vi "Create Icon Framework.vi"(10 "Template Glyph":picture, 11 "Layer name":string) -> (3 "Icon Framework out":refnum<class "Icon Framework.lvclass">)   [LabVIEW 2020, in "LabVIEW Icon API.lvlib"]
doc: "Create the Icon Framework (Template or Text class) class."
uses:
  <vilib>/LabVIEW Icon API/LabVIEW Icon API.lvlib
  <vilib>/LabVIEW Icon API/lv_icon/Classes/Icon Framework/Icon Framework.lvclass
  <vilib>/LabVIEW Icon API/lv_icon/Controls/Layer.ctl
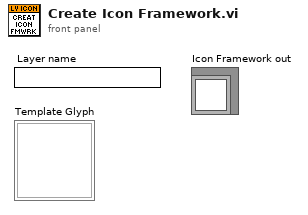
[diagram p1: front panel]
types:
  T1 = typedef "Layer.ctl" = cluster{"LayerIcon":picture, "LayerName":string, "Opacity":u8, "Visibility?":bool}
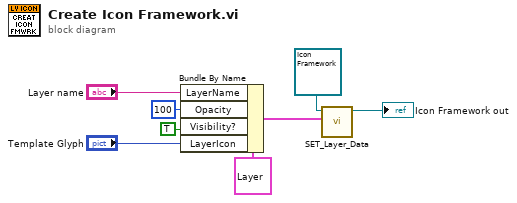
[diagram p0: block diagram]
diagram:
  n1 = Bundle By Name(cluster=T1 {"LayerIcon"=bytes[3102], "LayerName"="", "Opacity"=100, "Visibility?"=TRUE} ("Data"), "LayerName"="Layer name", "Opacity"=u8 100, "Visibility?"=TRUE, "LayerIcon"="Template Glyph") -> (w8:T1)
  n2 = call-dynamic "SET_Layer_Data.vi"("Data"=w8, "Layer.lvclass in"=refnum<class "Icon Framework.lvclass"> refnum ("lv_icon.lvlib:Icon Framework.lvclass")) -> ("Layer.lvclass out"=→"Icon Framework out":refnum<class "Icon Framework.lvclass">)  [unwired: 8 in, 1 out]
